vi "Connect.vi"(8 "error in":errorcluster, 11 "DMK33UP2000 in":refnum<class "DMK33UP2000.lvclass">) -> (0 "error out":errorcluster, 3 "DMK33UP2000 out":refnum<class "DMK33UP2000.lvclass">)   [LabVIEW 2018, in "DMK33UP2000.lvlib" / "DMK33UP2000.lvclass"]
uses:
  DMK33UP2000.lvclass
  <vilib>/vision/driver/IMAQdx.llb/IMAQdx Acquisition Mode.ctl
  <vilib>/vision/driver/NI_Vision_Acquisition_Software.lvlib
  builds/Camera.lvlibp/Camera.lvclass
  C:/Users/Ron.Dexter.LUMINARTECH/Desktop/builds/Camera.lvlibp/Camera.lvclass
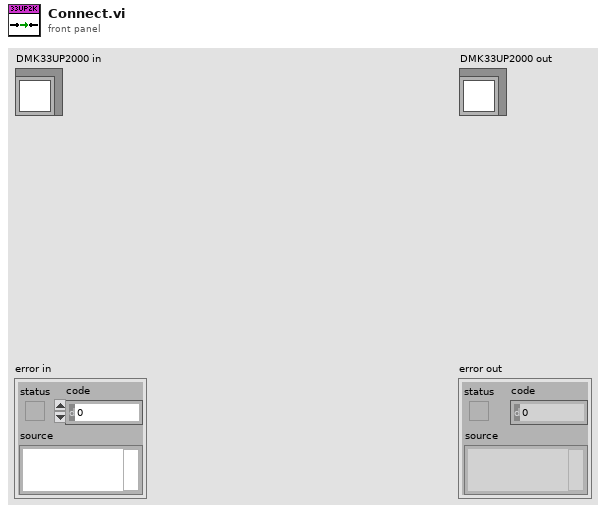
[diagram p1: front panel]
types:
  T1 = typedef "NI_Vision_Acquisition_Software.lvlib/IMAQdx Acquisition Mode.ctl" = enum32{"One Shot", "Continuous"}
  T2 = typedef "Camera.lvlibp/IMAQdx.ctl" = refnum<k21>
  T3 = typedef "IMAQdx.ctl" = refnum<k21>
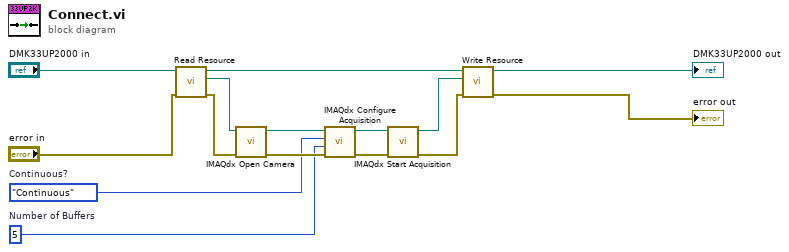
[diagram p0: block diagram]
diagram:
  w13 = u32 5  # Number of Buffers
  w1 = IMAQdx_Acquisition_Mode."Continuous"  # Continuous?
  n1 = call "Read Resource.vi"("error in (no error)"="error in", "Camera in"="DMK33UP2000 in") -> ("error out"=w8:errorcluster, "IMAQdx Session"=w7:T2, "Camera out"=w6:refnum<class "DMK33UP2000.lvclass">)  [unwired: 7 in]
  n2 = call <vilib>:"IMAQdx Open Camera.vi"("error in"=w8, "Session In"=w7) -> ("error out"=w14:errorcluster, "Session Out"=w15:T3)  [unwired: 8 in]
  n3 = call <vilib>:"IMAQdx Configure Acquisition.vi"("error in"=w14, "Number of Buffers"=w13, "Continuous?"=w1, "Session In"=w15) -> ("error out"=w11:errorcluster, "Session Out"=w12:T3)  [unwired: 6 in]
  n4 = call <vilib>:"IMAQdx Start Acquisition.vi"("error in"=w11, "Session In"=w12) -> ("error out"=w3:errorcluster, "Session Out"=w4:T3)  [unwired: 8 in]
  n5 = call "Write Resource.vi"("error in (no error)"=w3, "IMAQdx Session"=w4, "Camera in"=w6) -> ("error out"=→"error out":errorcluster, "Camera out"=→"DMK33UP2000 out":refnum<class "DMK33UP2000.lvclass">)  [unwired: 7 in]
